vi "RGB2Led.vi"(1 "B":u8, 2 "G":u8, 3 "R":u8) -> (0 "Colors [4]":cluster{u32, u32}[](array[cluster]))   [LabVIEW 2018]
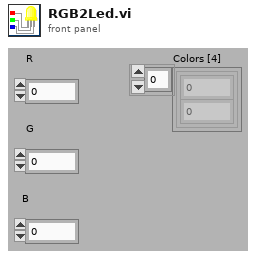
[diagram p1: front panel]
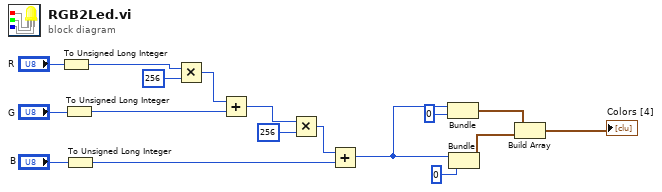
[diagram p0: block diagram]
diagram:
  n1 = To Unsigned Long Integer(number="R") -> (unsigned 32bit integer=w3:u32)
  n2 = To Unsigned Long Integer(number="G") -> (unsigned 32bit integer=w2:u32)
  n3 = To Unsigned Long Integer(number="B") -> (unsigned 32bit integer=w1:u32)
  n4 = Multiply(x=w3, y=u32 256) -> (x*y=w14:u32)
  n5 = Add(x=w14, y=w2) -> (x+y=w15:u32)
  n6 = Multiply(x=w15, y=u32 256) -> (x*y=w16:u32)
  n7 = Add(x=w16, y=w1) -> (x+y=w7:u32)
  n8 = Bundle(w7, "millisecond multiple"=u32 0) -> (w8:cluster{u32, "millisecond multiple":u32})  [unwired: 1 in]
  n9 = Bundle(w7, "millisecond multiple"=u32 0) -> (w9:cluster{u32, "millisecond multiple":u32})  [unwired: 1 in]
  n10 = Build Array(w8, w9) -> (→"Colors [4]":cluster{u32, "millisecond multiple":u32}[])
